vi "Add Item.vi"(5 "Path":path, 7 "error in":errorcluster, 8 "Path to start the search":path, 9 "Parent Tag":string, 10 "Tree In":refnum<vi>) -> (0 "error out":errorcluster, 2 "Folders Found":path[](array[path]), 3 "Tree Out":refnum<vi>)   [LabVIEW 2013, in "main.lvlib"]
doc: "This VI populates the tree control with the folders and their respective subfolders and files. \nIf Pattern to search control has a valid file type extension, only those files will be displayed."
uses:
  main.lvlib
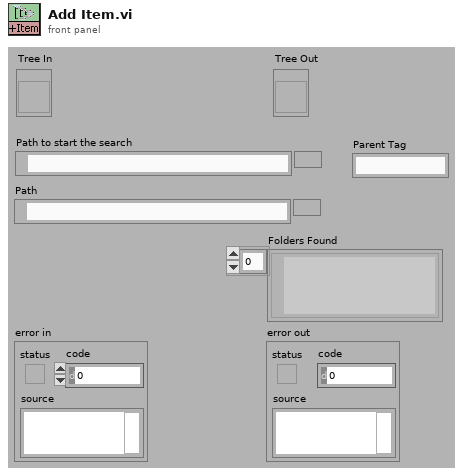
[diagram p1: front panel]
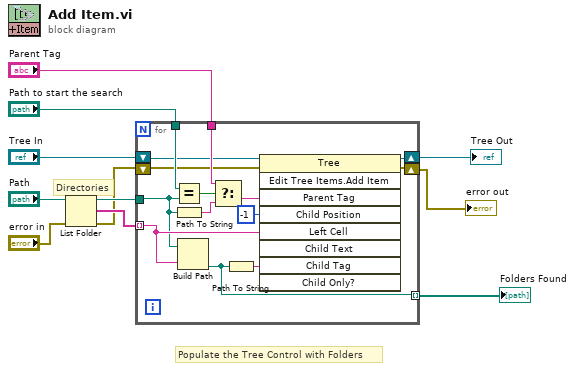
[diagram p0: block diagram]
diagram:
  # "Populate the Tree Control with Folders"
  # "Directories"
  n1 = List Folder(path="Path", error in="error in") -> (path out=w10:path, folder names=w6:string[], error out=w4:errorcluster)  [unwired: 2 in, 1 out]
  n2 = for {
    tunnel: w10 -> [w17]
    tunnel: [w23] -> w9 mode=indexing
    tunnel: w6 -> [w24] mode=indexing
    tunnel: "Parent Tag" -> [w19]
    tunnel: "Path to start the search" -> [w16]
    shift-right: [w14] -> w2
    shift-left: w4 -> [w13]
    shift-right: [w12] -> w1
    shift-left: "Tree In" -> [w15]
    n3 = Equal?(x=w16, y=w17) -> (x = y?=w21:bool)
    n4 = Path To String(path=w17) -> (string=w20:string)
    n5 = Build Path(base path=w17, name or relative path=w24) -> (appended path=w23:path)
    n6 = Select(t=w19, s=w21, f=w20) -> (s? t:f=w18:string)
    n7 = Path To String(path=w23) -> (string=w22:string)
    n8 = invoke on="Invoke Node" class="Tree" method="Edit Tree Items.Add Item"(reference=w15, error in=w13, "Parent Tag"=w18, "Child Position"=-1 ("Child Posn"), "Left Cell"=w24, "Child Tag"=w22) -> (reference out=w12:refnum<vi>, error out=w14:errorcluster)  [unwired: 3 in, 7 out]
  }
  "Folders Found" <- w9
  "error out" <- w2
  "Tree Out" <- w1
